vi "Meas Proc QWTB Parse Table.vi"(8 "error in":errorcluster, 11 "param table ref":refnum<vi>) -> (0 "error out":errorcluster, 3 "qwtb parameters":T1[](array[typedef]))   [LabVIEW 2018]
doc: "Parses string table into QWTB parameters. It takes each nonempty row header, extracts variable name and then scans through row of the table. If all values in the parameter's row matches numeric values it assumes it is numeric parameter. If not, it assumes it is string parameter."
uses:
  Meas Proc QWTB Algorithm Parameter Data.ctl
  <vilib>/regexp/Match Regular Expression.xnode
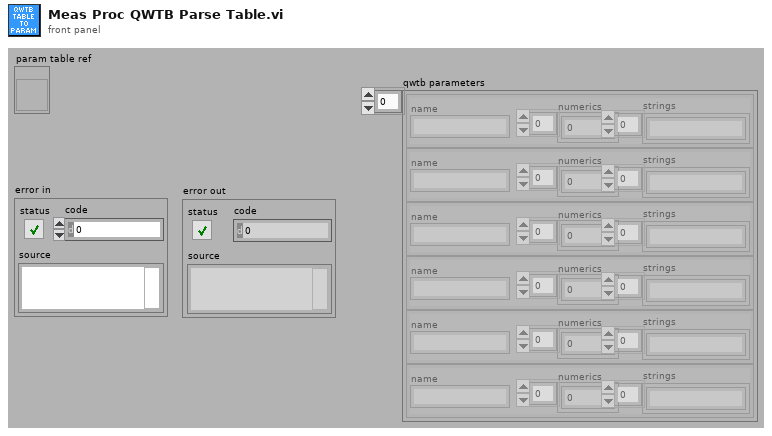
[diagram p1: front panel]
types:
  T1 = typedef "Meas Proc QWTB Algorithm Parameter Data.ctl" = cluster{"name":string, "numerics":dbl[], "strings":string[]}
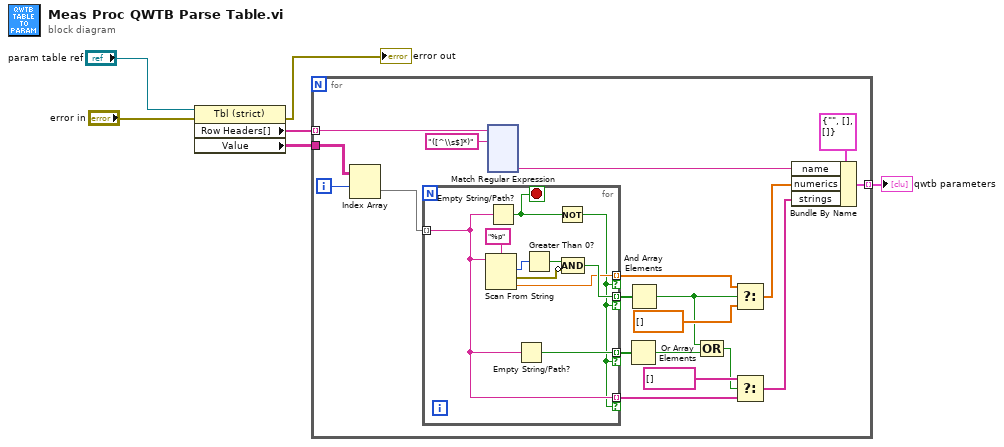
[diagram p0: block diagram]
diagram:
  n1 = property class="Tbl (strict)"(reference="param table ref", error in="error in") -> (error out=→"error out":errorcluster, "Row Headers[]"=w4:string[], "Value"=w3:string[][])  [unwired: 1 out]
  n2 = for {
    tunnel: w4 -> [w25] mode=indexing
    tunnel: w3 -> [w13]
    tunnel: [w14] -> w2 mode=indexing
    i -> [w12]
    n3 = Index Array(array=w13, index (row)=w12) -> (element=w11:string[])  [unwired: 1 in]
    n4 = for {
      tunnel: w11 -> [w29] mode=indexing
      tunnel: [w30] -> w20 mode=indexing if=w26
      tunnel: [w31] -> w21 mode=indexing if=w26
      tunnel: [w29] -> w17 mode=indexing if=w26
      tunnel: [w28] -> w8 mode=indexing if=w26
      stop <- w27 stop-if-true
      n5 = Scan From String(format string="%p", input string=w29) -> (offset past scan=w34:u32, error out=w32:errorcluster, output 1=w30:dbl)  [unwired: 3 in, 1 out]
      n6 = Empty String/Path?(string/path=w29) -> (empty?=w27:bool)
      n7 = Empty String/Path?(string/path=w29) -> (empty?=w28:bool)
      n8 = Greater Than 0?(x=w34) -> (x > 0?=w33:bool)
      n9 = Not(x=w27) -> (.not. x?=w26:bool)
      n10 = Compound Arithmetic op=AND(w33, invert w32) -> (w31:bool)
    }
    n11 = xnode "Match Regular Expression"("input string"=w25, "regular expression"="([^\\s$]*)") -> ("submatch 1"=w22:string)  [unwired: 4 in, 5 out]
    n12 = Or Array Elements(Boolean array=w8) -> (logical OR=w7:bool)
    n13 = And Array Elements(Boolean array=w21) -> (logical AND=w9:bool)
    n14 = Compound Arithmetic op=OR(w9, w7) -> (w10:bool)
    n15 = Select(t=w20, s=w9, f=dbl[] []) -> (s? t:f=w18:dbl[])
    n16 = Select(t=string[] [], s=w10, f=w17) -> (s? t:f=w15:string[])
    n17 = Bundle By Name(cluster=T1 {"name"="", "numerics"=[], "strings"=[]} ("qwtb parameter"), "name"=w22, "numerics"=w18, "strings"=w15) -> (w14:T1)
  }
  "qwtb parameters" <- w2
